vi "List Directory Recursive with Progress Bar Popup.vi"(6 "List only Top-Level files in llbs? (FALSE)":bool, 8 "error in (no error)":errorcluster, 9 "Treat llb files as directories? (FALSE)":bool, 10 "pattern":string, 11 "Path":path) -> (0 "error out":errorcluster, 1 "dir paths":path[](array[path]), 2 "file paths":path[](array[path]), 3 "dup Path":path)   [LabVIEW 2014]
doc: "Returns an array of strings listing the names of all files in directory path and its subfolders, filtering the file names array based upon the specified pattern. If \"Treat llb files as directories\" is TRUE, llb files will not show up in the \"file paths\" output, but thier contents will. If \"List only Top-level files in llbs?\" is TRUE, only top-level llb contents will show up in the \"file paths\" output."
uses:
  <userlib>/_OpenG.lib/file/file.llb/Build Path - File Names Array__ogtk.vi
  <userlib>/_OpenG.lib/array/array.llb/Filter 1D Array (Path)__ogtk.vi
  <userlib>/_OpenG.lib/array/array.llb/Remove Duplicates from 1D Array (Path)__ogtk.vi
panel:
  # "[OpenG VI Tags] ***Do Not Remove***"
  # "List Recursive.vi\n\nGets an array of all files in dir and its sub-dir's\n\nPlease visit http://www.OpenG.org to learn about the\nOpen Source LabVIEW software movement.\n\nNOTICE -- YOU MUST LEAVE THIS NOTICE IN PLACE.  PER THE TERMS OF THE LICENSE BELOW, YOU MAY SUBLICENSE THIS SOFTWARE \nIN ANY WAY THAT DOES NOT CONFLICT WITH THIS LICENSE.\n\n### BSD License (http://www.opensource.org/licenses/bsd-license.php) Begin ###\n \nCopyright (c) 2002-2006, Jim Kring <jim@jimkring.com>\nCopyright (c) 2002, Cal-Bay Systems, Inc. <info@calbay.com>\n\nAll rights reserved.\n\nRedistribution and use in source and binary forms, with or without modification, are permitted provided that the following conditions are met:\n\n    * Redistributions of source code must retain the above copyright notice, this list of conditions and the following disclaimer.\n    * Redistributions in binary form must reproduce the above copyright notice, this list of conditions and the following disclaimer in the \n       documentation and/or other materials provided with the distribution.\n    * Neither the name of SciWare, James Kring, Inc., nor the names of its contributors may be used to endorse or promote products derived \n       from this software without specific prior written permission.\n\nTHIS SOFTWARE IS PROVIDED BY THE COPYRIGHT HOLDERS AND CONTRIBUTORS \"AS IS\" AND ANY EXPRESS OR IMPLIED WARRANTIES, \nINCLUDING, BUT NOT LIMITED TO, THE IMPLIED WARRANTIES OF MERCHANTABILITY AND FITNESS FOR A PARTICULAR PURPOSE ARE \nDISCLAIMED. IN NO EVENT SHALL THE COPYRIGHT OWNER OR CONTRIBUTORS BE LIABLE FOR ANY DIRECT, INDIRECT, INCIDENTAL,\n SPECIAL, EXEMPLARY, OR CONSEQUENTIAL DAMAGES (INCLUDING, BUT NOT LIMITED TO, PROCUREMENT OF SUBSTITUTE GOODS OR \nSERVICES; LOSS OF USE, DATA, OR PROFITS; OR BUSINESS INTERRUPTION) HOWEVER CAUSED AND ON ANY THEORY OF LIABILITY, \nWHETHER IN CONTRACT, STRICT LIABILITY, OR TORT (INCLUDING NEGLIGENCE OR OTHERWISE) ARISING IN ANY WAY OUT OF THE USE \nOF THIS SOFTWARE, EVEN IF ADVISED OF THE POSSIBILITY OF SUCH DAMAGE.\n\n### BSD License End ###"
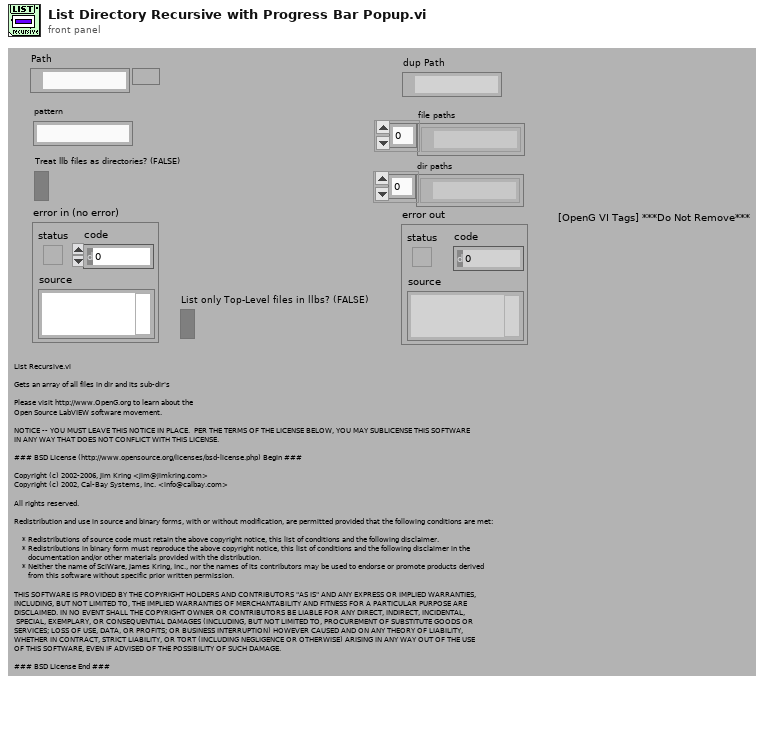
[diagram p1: front panel]
types:
  T1 = typedef "Librarian File Info Out.ctl" = cluster{"creation date":u32, "last mod date":u32, "type":string, "creator":string, "LV version":i32, "size":i32, "top level":bool}
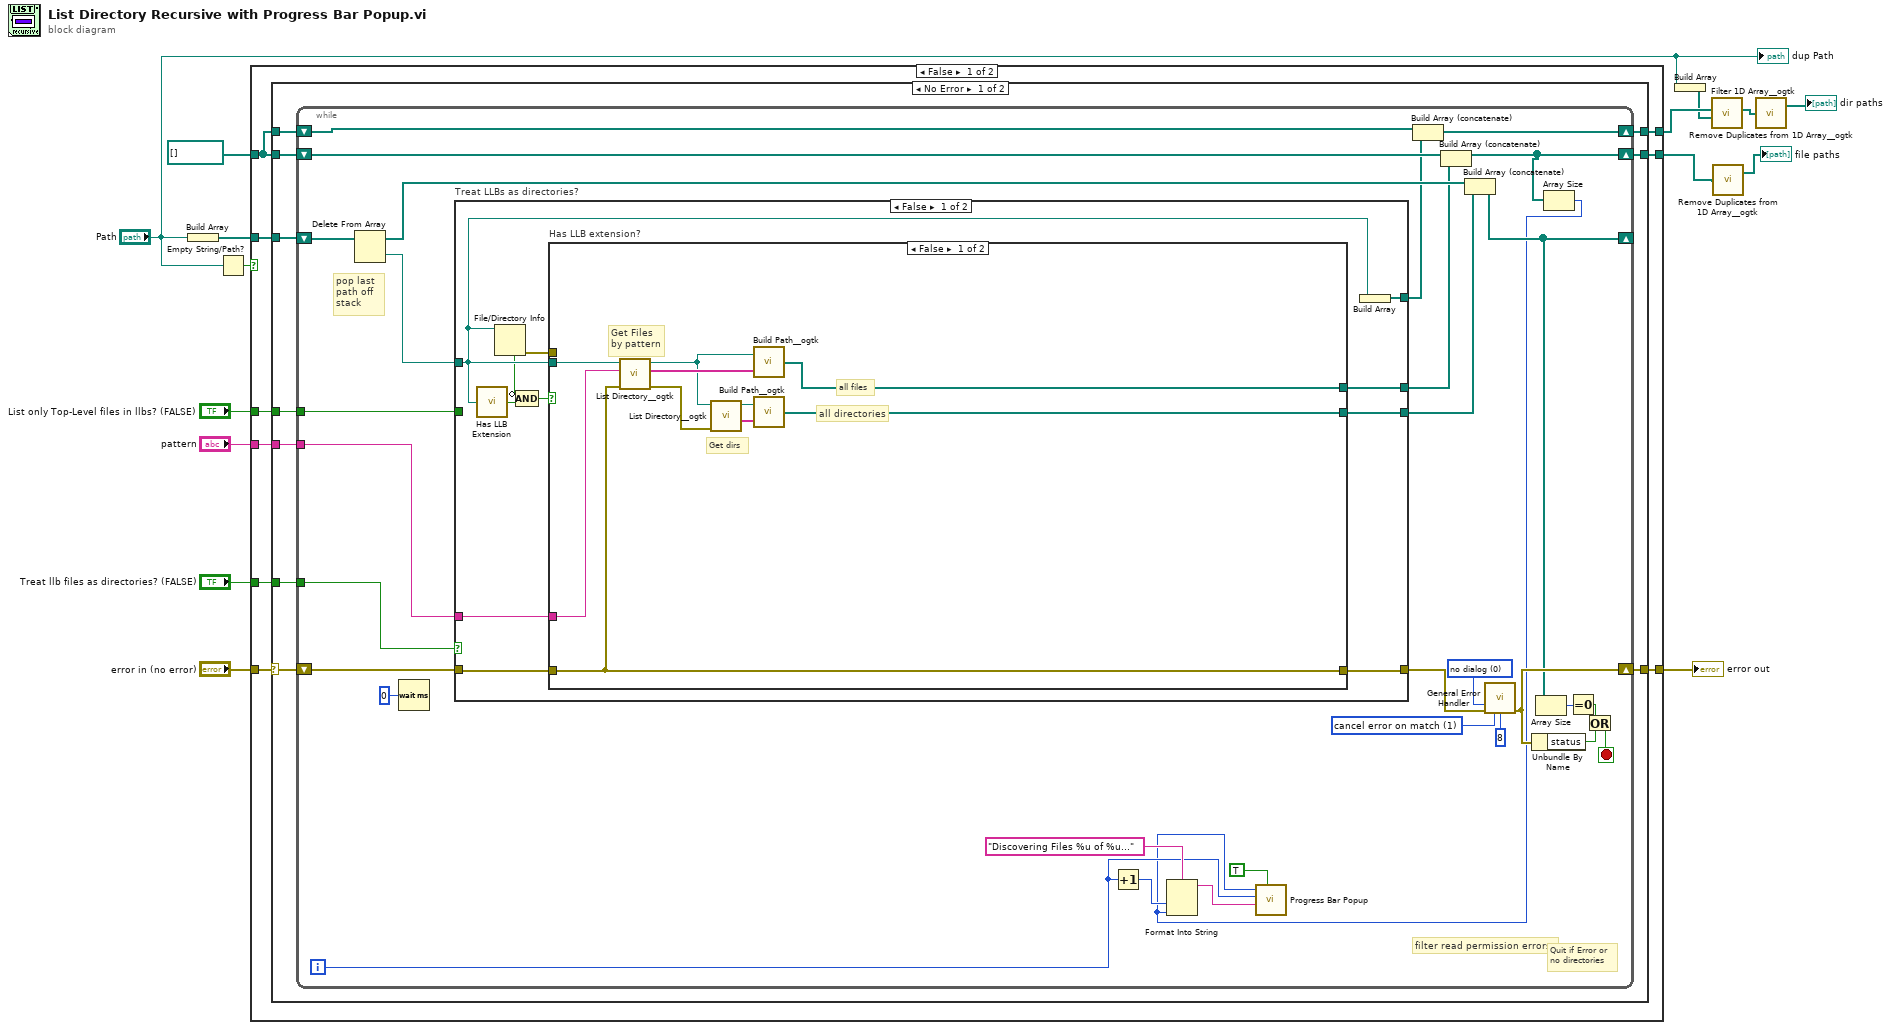
[diagram p0: block diagram]
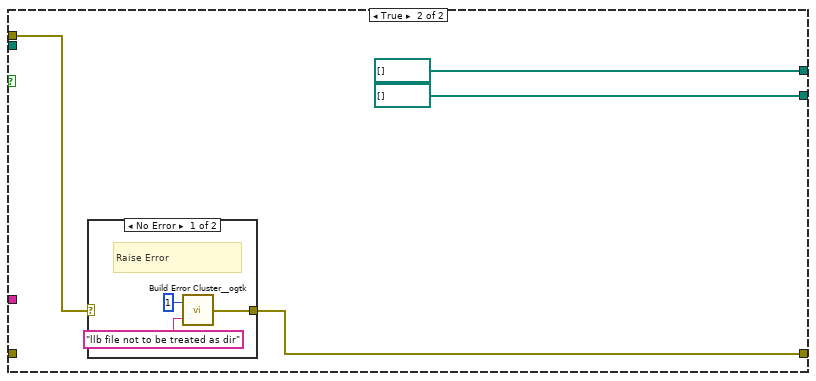
[diagram p2: hidden frame]
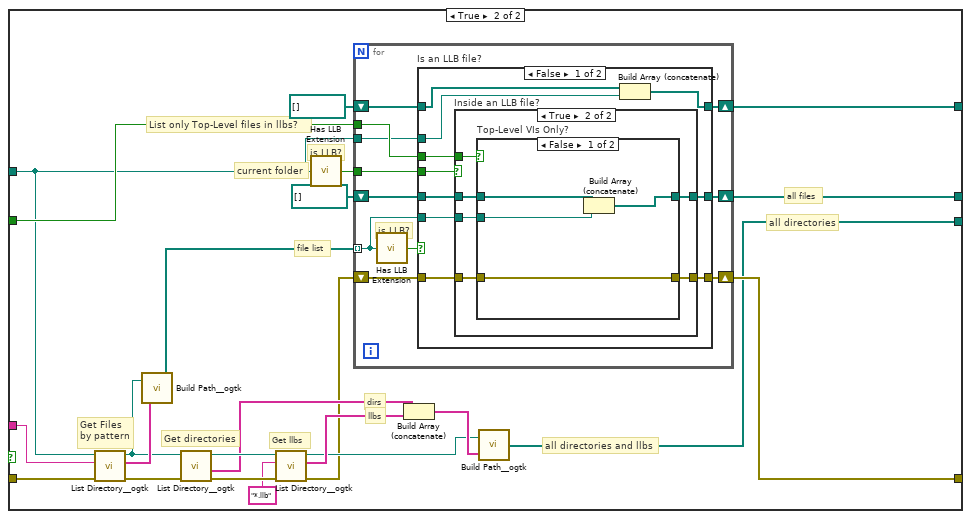
[diagram p4: hidden frame]
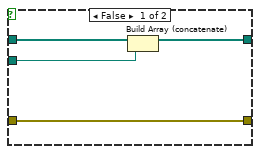
[diagram p5: hidden frame]
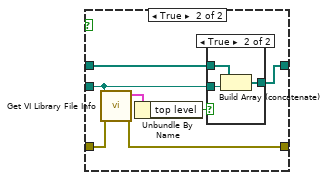
[diagram p6: hidden frame]
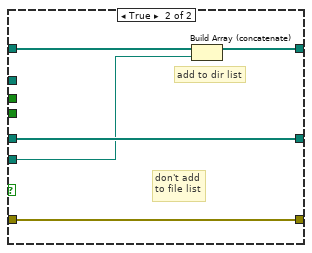
[diagram p8: hidden frame]
diagram:
  n1 = Build Array("Path") -> (w14:path[])
  n2 = Empty String/Path?(string/path="Path") -> (empty?=w8:bool)
  n3 = case shown="False" w8 {
    tunnel: [w24 w172] -> w15
    tunnel: w14 -> [w23 _]
    tunnel: path[] [] ("Array Constant") -> [w22 w173]
    tunnel: [w21 w173] -> w4
    tunnel: "pattern" -> [w20 _]
    tunnel: "Treat llb files as directories? (FALSE)" -> [w19 _]
    tunnel: "List only Top-Level files in llbs? (FALSE)" -> [w18 _]
    tunnel: "error in (no error)" -> [w17 w172]
    tunnel: [w16 w173] -> w7
    frame False {
      n4 = case shown="No Error" w17 {
        selector: w17 -> [w27 w171]
        tunnel: [w34 w171] -> w24
        tunnel: w23 -> [w33 _]
        tunnel: w22 -> [w32 w170]
        tunnel: [w31 w170] -> w21
        tunnel: w20 -> [w30 _]
        tunnel: w19 -> [w29 _]
        tunnel: w18 -> [w28 _]
        tunnel: w22 -> [w26 w169]
        tunnel: [w25 w169] -> w16
        frame No Error {
          n5 = while {
            shift-right: [w46] -> _
            shift-left: w33 -> [w60]
            shift-right: [w58] -> w34
            shift-left: w27 -> [w53]
            shift-right: [w36] -> w31
            shift-left: w32 -> [w59]
            tunnel: w30 -> [w52]
            tunnel: w29 -> [w47]
            tunnel: w28 -> [w48]
            shift-right: [w44] -> w25
            shift-left: w26 -> [w43]
            i -> [w37]
            stop <- w61 stop-if-true
            w55 = u16 0 items=["no dialog", "OK message", "continue or stop message"] ("type of dialog (OK msg:1)")
            w57 = 1 items=["no exception", "cancel error on match", "set error on match"] ("[exception action] (none:0)")
            # "filter read permission errors"
            # "pop last path off stack"
            # "Quit if Error or no directories"
            n6 = Delete From Array(array=w60) -> (deleted portion=w65:path, array with subset deleted=w50:path[])  [unwired: 2 in]
            n7 = Wait (ms)(milliseconds to wait=u32 0) -> ()  [unwired: 1 out]
            n8 = case "Treat LLBs as directories?" shown="False" w47 {
              tunnel: w65 -> [w70 w96]
              tunnel: w53 -> [w76 w116]
              tunnel: [w75 w100] -> w45
              tunnel: w52 -> [w74 w117]
              tunnel: w48 -> [_ w102]
              tunnel: [w72 w99] -> w51
              tunnel: [w73 w98] -> w49
              tunnel: [w71 w95] -> w42
              frame False {
                n9 = call <vilib>:"Has LLB Extension.vi"("path"=w70) -> ("path to VI library?"=w69:bool)
                n10 = File/Directory Info(path=w70) -> (directory=w67:bool, error out=w66:errorcluster)  [unwired: 1 in, 5 out]
                n11 = Compound Arithmetic op=AND(invert w67, w69) -> (w68:bool)
                n12 = case "Has LLB extension?" shown="False" w68 {
                  tunnel: w76 -> [w83 _]
                  tunnel: [w83 w88] -> w75
                  tunnel: w70 -> [w84 _]
                  tunnel: w74 -> [w86 _]
                  tunnel: [w82 path[] [] ("appended path")] -> w73
                  tunnel: [w77 path[] [] ("appended path")] -> w72
                  tunnel: w66 -> [_ w87]
                  frame False {
                    # "Get dirs"
                    # "all directories"
                    # "all files"
                    # "Get Files\nby pattern"
                    n13 = call <userlib>:"List Directory__ogtk.vi"("error in (no error)"=w83, "pattern"=w86, "directory path"=w84) -> ("error out"=w81:errorcluster, "file names"=w85:string[], "dup directory path"=w80:path)  [unwired: 1 in, 1 out]
                    n14 = call <userlib>:"List Directory__ogtk.vi"("error in (no error)"=w81, "directory path"=w80) -> ("directory names"=w79:string[], "dup directory path"=w78:path)  [unwired: 2 in, 2 out]
                    n15 = call-poly <userlib>:"Build Path__ogtk.vi"("name or relative path"=w85, "base path"=w80) -> ("appended path"=w82:path[])
                    n16 = call-poly <userlib>:"Build Path__ogtk.vi"("name or relative path"=w79, "base path"=w78) -> ("appended path"=w77:path[])
                  }
                  frame True {
                    n17 = case shown="No Error" w87 {
                      selector: w87 -> [_ w94]
                      tunnel: [w91 w94] -> w88
                      frame No Error {
                        # "Raise Error"
                        n18 = call <userlib>:"Build Error Cluster__ogtk.vi"("String to Prepend to source (\"\")"="llb file not to be treated as dir" ("String to Prepend to source (\"\")"), "code"=1) -> ("error out"=w91:errorcluster)
                      }
                      frame Error {
                      }
                    }
                  }
                }
                n19 = Build Array(w70) -> (w71:path[])
              }
              frame True {
                # "all directories"
                # "all files"
                # "List only Top-Level files in llbs?"
                # "all directories and llbs"
                # "llbs"
                # "dirs"
                # "file list"
                # "is LLB?"
                # "current folder"
                # "Get llbs"
                # "Get directories"
                # "Get Files\nby pattern"
                n20 = call <userlib>:"List Directory__ogtk.vi"("error in (no error)"=w116, "pattern"=w117, "directory path"=w96) -> ("error out"=w105:errorcluster, "file names"=w115:string[], "dup directory path"=w104:path)  [unwired: 1 in, 1 out]
                n21 = call-poly <userlib>:"Build Path__ogtk.vi"("name or relative path"=w115, "base path"=w104) -> ("appended path"=w114:path[])
                n22 = call <userlib>:"List Directory__ogtk.vi"("error in (no error)"=w105, "directory path"=w104) -> ("error out"=w112:errorcluster, "directory names"=w108:string[], "dup directory path"=w109:path)  [unwired: 2 in, 1 out]
                n23 = call <userlib>:"List Directory__ogtk.vi"("error in (no error)"=w112, "pattern"="*.llb", "directory path"=w109) -> ("error out"=w101:errorcluster, "file names"=w110:string[], "dup directory path"=w106:path)  [unwired: 1 in, 1 out]
                n24 = call <vilib>:"Has LLB Extension.vi"("path"=w96) -> ("path to VI library?"=w103:bool)
                n25 = for {
                  tunnel: w114 -> [w127] mode=indexing
                  shift-right: [w126] -> w98
                  shift-left: path[] [] -> [w125]
                  tunnel: w103 -> [w124]
                  tunnel: w102 -> [w123]
                  shift-right: [w121] -> w100
                  shift-left: w101 -> [w122]
                  shift-right: [w119] -> w95
                  shift-left: path[] [] -> [w120]
                  tunnel: w96 -> [w118]
                  # "is LLB?"
                  n26 = call <vilib>:"Has LLB Extension.vi"("path"=w127) -> ("path to VI library?"=w128:bool)
                  n27 = case "Is an LLB file?" shown="False" w128 {
                    tunnel: w127 -> [w135 w165]
                    tunnel: [w134 w168] -> w126
                    tunnel: w125 -> [w136 w168]
                    tunnel: w124 -> [w138 _]
                    tunnel: w123 -> [w137 _]
                    tunnel: w122 -> [w133 w167]
                    tunnel: [w132 w167] -> w121
                    tunnel: w120 -> [w131 w166]
                    tunnel: [w130 w164] -> w119
                    tunnel: w118 -> [w129 _]
                    frame False {
                      n28 = case "Inside an LLB file?" shown="True" w138 {
                        tunnel: w137 -> [_ w148]
                        tunnel: w136 -> [w142 w147]
                        tunnel: w135 -> [w141 w146]
                        tunnel: [w140 w145] -> w134
                        tunnel: w133 -> [w139 w144]
                        tunnel: [w139 w143] -> w132
                        frame False {
                          n29 = Build Array (concatenate)(w142, w141) -> (w140:path[])
                        }
                        frame True {
                          n30 = case "Top-Level VIs Only?" shown="False" w148 {
                            tunnel: w146 -> [w151 w153]
                            tunnel: w147 -> [w152 w159]
                            tunnel: [w150 w158] -> w145
                            tunnel: w144 -> [w149 w156]
                            tunnel: [w149 w155] -> w143
                            frame False {
                              n31 = Build Array (concatenate)(w152, w151) -> (w150:path[])
                            }
                            frame True {
                              n32 = call <vilib>:"Get VI Library File Info.vi"("error in (no error)"=w156, "path"=w153) -> ("error out"=w155:errorcluster, "file information"=w154:T1)  [unwired: 8 in]
                              n33 = Unbundle By Name(w154) -> ("top level"=w157:bool)
                              n34 = case shown="True" w157 {
                                tunnel: w159 -> [w160 w163]
                                tunnel: w153 -> [_ w162]
                                tunnel: [w160 w161] -> w158
                                frame False {
                                }
                                frame True {
                                n35 = Build Array (concatenate)(w163, w162) -> (w161:path[])
                                }
                              }
                            }
                          }
                        }
                      }
                      n36 = Build Array (concatenate)(w131, w129) -> (w130:path[])
                    }
                    frame True {
                      # "add to dir list"
                      # "don't add\nto file list"
                      n37 = Build Array (concatenate)(w166, w165) -> (w164:path[])
                    }
                  }
                }
                n38 = Build Array (concatenate)(w108, w110) -> (w107:string[])
                n39 = call-poly <userlib>:"Build Path__ogtk.vi"("name or relative path"=w107, "base path"=w106) -> ("appended path"=w99:path[])
              }
            }
            n40 = Increment(x=w37) -> (x+1=w38:i32)
            n41 = Build Array (concatenate)(w43, w42) -> (w44:path[])
            n42 = Build Array (concatenate)(w59, w49) -> (w36:path[])
            n43 = Build Array (concatenate)(w50, w51) -> (w46:path[])
            n44 = call <vilib>:"General Error Handler.vi"("type of dialog (OK msg:1)"=w55, "error in (no error)"=w45, "[exception action] (none:0)"=w57, "[exception code]"=8) -> ("error out"=w58:errorcluster)  [unwired: 7 in, 4 out]
            n45 = Unbundle By Name(w58) -> ("status"=w63:bool)
            n46 = Array Size(array=w46) -> (size(s)=w64:i32)
            n47 = Array Size(array=w36) -> (size(s)=w35:i32)
            n48 = Format Into String(format string="Discovering Files %u of %u..." ("Message (Please Wait...)"), w38, w35) -> (resulting string=w40:string)  [unwired: 2 in, 1 out]
            n49 = call "Progress Bar Popup.vi"("Abort visible? (T)"=TRUE, "Message (Please Wait...)"=w40, "Current Iteration"=w37, "Total Iterations"=w35) -> ()  [unwired: 7 in, 1 out]
            n50 = Equal To 0?(x=w64) -> (x = 0?=w62:bool)
            n51 = Or(x=w62, y=w63) -> (x .or. y?=w61:bool)
          }
        }
        frame Error {
        }
      }
    }
    frame True {
    }
  }
  "error out" <- w15
  n52 = Build Array("Path") -> (w5:path[])
  n53 = call-poly <userlib>:"Filter 1D Array__ogtk.vi"("items to filter"=w5, "array"=w7) -> ("filtered array"=w2:path[])  [unwired: 4 in, 1 out]
  n54 = call-poly <userlib>:"Remove Duplicates from 1D Array__ogtk.vi"("Input Array"=w4) -> ("Output Array"=→"file paths":path[])  [unwired: 1 out]
  n55 = call-poly <userlib>:"Remove Duplicates from 1D Array__ogtk.vi"("Input Array"=w2) -> ("Output Array"=→"dir paths":path[])  [unwired: 1 out]
  "dup Path" <- "Path"
